vi "toJSON.vi"(8 "error in (no error)":errorcluster, 11 "tBSON_I64 in":refnum<class "tBSON_I64.lvclass">) -> (0 "error out":errorcluster, 2 "JSON":string, 3 "tBSON_I64 out":refnum<class "tBSON_I64.lvclass">)   [LabVIEW 2013, in "BSON.lvlib" / "tBSON_I64.lvclass"]
uses:
  tBSON_I64.lvclass
  tBSONElement/tBSONElement.lvclass
  getValue.vi
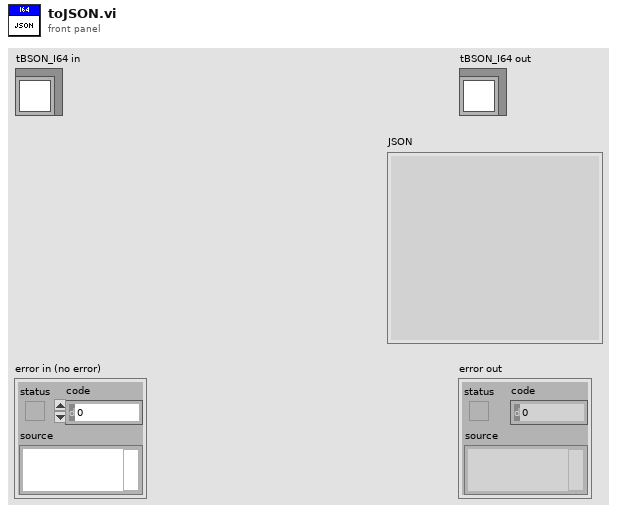
[diagram p1: front panel]
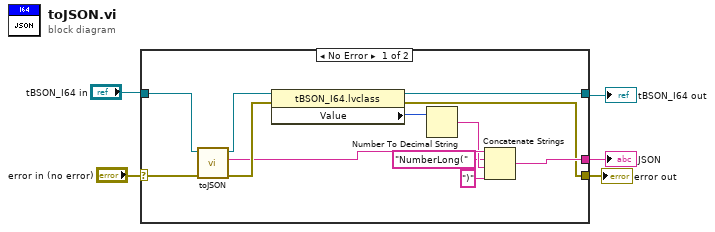
[diagram p0: block diagram]
diagram:
  n1 = case shown="No Error" "error in (no error)" {
    selector: "error in (no error)" -> [w16 w18]
    tunnel: "tBSON_I64 in" -> [w17 w19]
    tunnel: [w11 w18] -> w2
    tunnel: [w10 w19] -> w4
    tunnel: [w12 _] -> w3
    frame No Error {
      n2 = call-parent "toJSON.vi"("error in (no error)"=w16, "tBSONElement in"=w17) -> ("error out"=w14:errorcluster, "JSON"=w9:string, "tBSONElement out"=w15:refnum<class "tBSON_I64.lvclass">)  [unwired: 7 in]
      n3 = property class="tBSON_I64.lvclass"(reference=w15, error in=w14) -> (reference out=w10:refnum<class "tBSON_I64.lvclass">, error out=w11:errorcluster, "Value"=w13:i64)
      n4 = Number To Decimal String(number=w13) -> (decimal integer string=w8:string)  [unwired: 1 in]
      n5 = Concatenate Strings(w9, "NumberLong(" ("string"), w8, ")" ("string")) -> (w12:string)
    }
    frame Error {
    }
  }
  "error out" <- w2
  "tBSON_I64 out" <- w4
  "JSON" <- w3
